vi "StartUp Sequence Open Loop Rev 1.5.vi"() -> ()   [LabVIEW 2017]
panel:
  out "Requested RPM":i32
  out "Waveform Chart":cluster{i32, i32}(graph)
  in  "Set RPM":string
  out "Pump Value 2":string
  in  "Soft Shut Off":bool
  out "Pump Value 1":string
  in  "Send RPM":bool
  in  "Send Command":bool
  in  "Custom Command":string
  out "Startup Success":bool
  in  "Output File":path
  in  "Shut Off":bool
  out "ECU COM Port Out":refnum<visa-resource-name>
  out "Throttle Position":string
  out "Turbine RPM":string
  out "Turbine Temp":string
  out "Error Out":errorcluster
  in  "Error In":errorcluster
  in  "ECU COM Port":refnum<visa-resource-name>
  out "Turbine State":string
  in  "Strt Sqnc":bool
  # "Note: save to a .csv file"
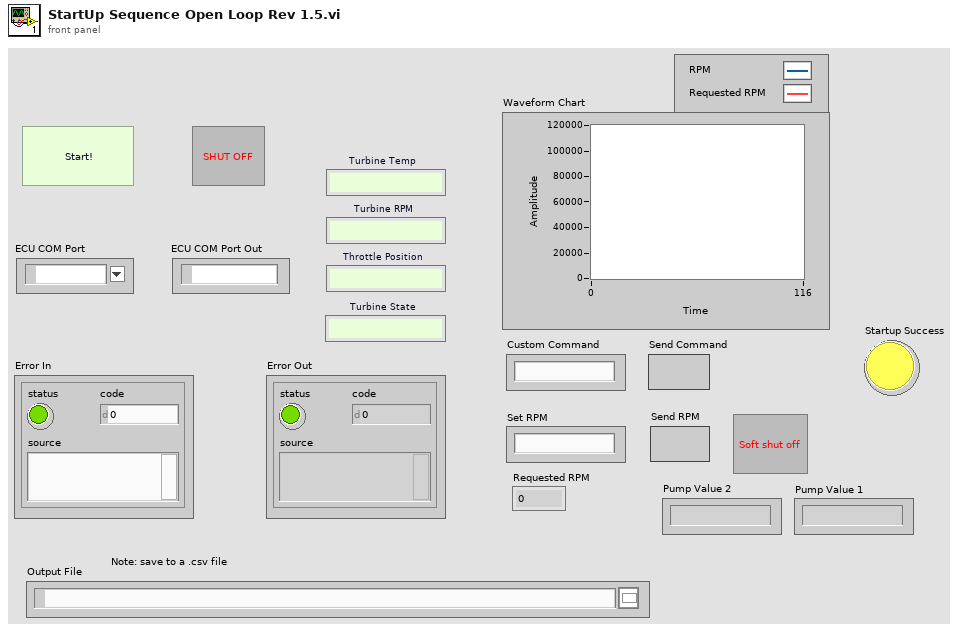
[diagram p1: front panel]
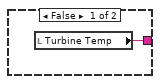
[diagram p4: hidden frame]
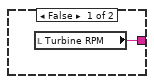
[diagram p5: hidden frame]
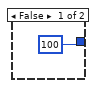
[diagram p7: hidden frame]
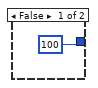
[diagram p8: hidden frame]
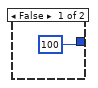
[diagram p9: hidden frame]
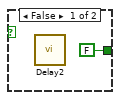
[diagram p11: hidden frame]
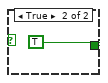
[diagram p12: hidden frame]
diagram:
  w15 = 21 ("Pulse Width")
  w16 = 160 ("Voltage")
  w21 = 16 ("Pulse Width")
  w22 = 160 ("Voltage")
  w12 = 255 ("y")
  w13 = 80 ("y")
  # "Disengage Starter Motor"
  # "Starter Motor 55%"
  # "Start button is inside a while loop that doesn't progess until True"
  # "Fuel Pump Mode 2"
  # "GlowPlugOff"
  # "Start Up\nFuelPumpMode 1"
  # "BurnerValveIgnitionPercent"
  # "If False, each Case structure is set\nto an arbitrary Delay time of 0.2 s"
  # "Each Stage is inside a while loop so that \nthe sequence doesn't progress until True"
  n1 = call "Initialize Com Port.vi"("Error In"="Error In", "ECU COM Port"="ECU COM Port") -> ("Error Out"=w36:errorcluster, "ECU COM Port Out"=w35:refnum<visa-resource-name>)  [unwired: 8 in]
  n2 = while {
    tunnel: w36 -> [w97]
    tunnel: [w97] -> w34
    stop <- "Strt Sqnc" stop-if-true
  }
  n3 = call "Initialize Output File.vi"("error in (no error)"=w34, "File Path Control"="Output File") -> ("error out"=w11:errorcluster)  [unwired: 9 in]
  n4 = flat-sequence {
    tunnel: w11 -> [w99]
    tunnel: [w99] -> w26
    frame #0 {
      n5 = local write "Strt Sqnc"(FALSE ("Strt Sqnc")) -> ()
    }
  }
  n6 = flat-sequence {
    tunnel: [w102] -> w10
    tunnel: w11 -> [w102]
    frame #0 {
      w101 = "0" ("Pump Value 1")
      n7 = local write "Pump Value 2"(w101) -> ()
      n8 = local write "Pump Value 1"(w101) -> ()
    }
  }
  n9 = while {
    tunnel: w10 -> [w123]
    tunnel: w35 -> [w122]
    tunnel: "Output File" -> [w119]
    stop <- w118 continue-if-true
    n10 = call "Get Engine Update.vi"("Error In"=w123, "ECU COM Port"=w122) -> ("Error Out"=w120:errorcluster, "Temperature"=w111:string, "RPMs"=w115:string, "ECU COM Port Out"=w117:refnum<visa-resource-name>)  [unwired: 6 in]
    n11 = call "Time Delay4"() -> ()  [unwired: 11 in, 1 out]
    n12 = call "Safety Check.vi"("Temperature"=w111, "RPMs"=w115) -> ("Safe?"=w118:bool)  [unwired: 9 in]
    n13 = Not Equal?(x=w115, y="") -> (x != y?=w113:bool)
    n14 = Not Equal?(x=w111, y="") -> (x != y?=w110:bool)
    n15 = case shown="False" w118 {
      selector: w118 -> [w128 w130]
      tunnel: w117 -> [w129 _]
      tunnel: [w128 w130] -> w116
      frame False {
        n16 = call "Emergency Shutoff.vi"("ECU COM Port"=w129) -> ()  [unwired: 9 in, 2 out]
      }
      frame True {
      }
    }
    n17 = case shown="True" w113 {
      tunnel: w115 -> [_ w127]
      tunnel: [w126 w127] -> w107
      frame False {
        n18 = local read "Turbine RPM"() -> (w126:string)
      }
      frame True {
        "Turbine RPM" <- w127
      }
    }
    n19 = case shown="True" w110 {
      tunnel: w111 -> [_ w125]
      tunnel: [w124 w125] -> w106
      frame False {
        n20 = local read "Turbine Temp"() -> (w124:string)
      }
      frame True {
        "Turbine Temp" <- w125
      }
    }
    n21 = Not(x=w116) -> (.not. x?=w121:bool)
    n22 = Stop(stop? (T)=w121) -> ()
    n23 = local read "Requested RPM"() -> (w104:i32)
    n24 = local read "Pump Value 2"() -> (w108:string)
    n25 = local read "Pump Value 1"() -> (w109:string)
    n26 = Decimal String To Number(string=w107) -> (number=w105:i32)  [unwired: 2 in, 1 out]
    n27 = Bundle(w105, "Requested RPM"=w104) -> (→"Waveform Chart":cluster{i32, "Requested RPM":i32})  [unwired: 1 in]
    n28 = call "Write Data to Output File.vi"("Pump Value 2"=w108, "Pump Value 1"=w109, "Error In"=w120, "Temperature"=w106, "RPM"=w107, "File Path Control"=w119) -> ()  [unwired: 5 in, 1 out]
  }
  n29 = while {
    tunnel: w35 -> [w132]
    tunnel: w36 -> [_]
    stop <- FALSE stop-if-true
    n30 = case shown="True" "Send Command" {
      tunnel: "Custom Command" -> [_ w136]
      tunnel: w132 -> [_ w135]
      frame False {
      }
      frame True {
        n31 = call "Time Delay3"() -> ()  [unwired: 11 in, 1 out]
        n32 = VISA Write(VISA resource name=w135, write buffer=w136) -> ()  [unwired: 1 in, 3 out]
      }
    }
  }
  n33 = flat-sequence {
    tunnel: w26 -> [_]
    frame #0 {
      n34 = local write "Turbine State"("Initializing Motor") -> ()
    }
  }
  n35 = while {
    tunnel: ["Shut Off"] -> w94
    tunnel: "ECU COM Port" -> [w138]
    stop <- "Shut Off" stop-if-true
    # "Turns off each individual component"
    n36 = case shown="True" "Shut Off" {
      tunnel: w138 -> [_ w142]
      frame False {
      }
      frame True {
        n37 = call "Emergency Shutoff.vi"("ECU COM Port"=w142) -> ("Error Out"=w141:errorcluster)  [unwired: 9 in, 1 out]
        n38 = local write "Output File"(path "" ("Output File")) -> ()
        n39 = flat-sequence {
          tunnel: w141 -> [w143]
          tunnel: [w143] -> _
          frame #0 {
            n40 = local write "Strt Sqnc"(FALSE ("Strt Sqnc")) -> ()
          }
        }
      }
    }
  }
  n41 = call "Set Glow Plug Duty Cycle.vi"("Error In"=w26, "Duty Cycle"=6, "ECU COM Port"=w35) -> ("Error Out"=w86:errorcluster, "ECU COM Port Out"=w83:refnum<visa-resource-name>)  [unwired: 7 in]
  n42 = call "Delay"("error in (no error)"=w86) -> ("error out"=w85:errorcluster)  [unwired: 10 in]
  n43 = call "Set Glow Plug Duty Cycle.vi"("Error In"=w85, "Duty Cycle"=19, "ECU COM Port"=w83) -> ("Error Out"=w84:errorcluster, "ECU COM Port Out"=w79:refnum<visa-resource-name>)  [unwired: 7 in]
  n44 = call "Delay"("error in (no error)"=w84) -> ("error out"=w80:errorcluster)  [unwired: 10 in]
  n45 = call "Set Starter Motor Duty Cycle.vi"("Error In"=w80, "Duty Cycle"=6, "ECU COM Port"=w79) -> ("Error Out"=w78:errorcluster, "ECU COM Port Out"=w76:refnum<visa-resource-name>)  [unwired: 7 in]
  n46 = call "Set Glow Plug Duty Cycle.vi"("Error In"=w78, "Duty Cycle"=15, "ECU COM Port"=w76) -> ("Error Out"=w77:errorcluster, "ECU COM Port Out"=w72:refnum<visa-resource-name>)  [unwired: 7 in]
  n47 = call "Delay"("error in (no error)"=w77) -> ("error out"=w74:errorcluster)  [unwired: 10 in]
  n48 = call "Set Starter Motor Duty Cycle.vi"("Error In"=w74, "Duty Cycle"=4, "ECU COM Port"=w72) -> ("Error Out"=w73:errorcluster, "ECU COM Port Out"=w71:refnum<visa-resource-name>)  [unwired: 7 in]
  n49 = call "Delay"("error in (no error)"=w73) -> ("error out"=w95:errorcluster)  [unwired: 10 in]
  n50 = Stop(stop? (T)=w94) -> ()
  n51 = while {
    tunnel: w95 -> [w147]
    tunnel: w71 -> [w146]
    tunnel: [w146] -> w24
    tunnel: [w147] -> w96
    stop <- w150 stop-if-true
    n52 = local read "Turbine RPM"() -> (w145:string)
    n53 = Decimal String To Number(string=w145) -> (number=w149:i32)  [unwired: 2 in, 1 out]
    n54 = Greater Or Equal?(x=w149, y=3300) -> (x >= y?=w151:bool)
    n55 = case shown="True" w151 {
      tunnel: [FALSE TRUE] -> w150
      frame False {
        n56 = call "Delay2"() -> ()  [unwired: 11 in, 1 out]
      }
      frame True {
      }
    }
  }
  n57 = flat-sequence {
    tunnel: w95 -> [_]
    frame #0 {
      n58 = local write "Turbine State"("Stage1 Check RPM") -> ()
    }
  }
  n59 = call "CmdSeparator7"("error in (no error)"=w96) -> ("error out"=w20:errorcluster)  [unwired: 10 in]
  n60 = call "Set Pump Fow Rate.vi"("Error In"=w20, "Pulse Width"=w21, "Voltage"=w22, "ECU COM Port"=w24) -> ("Error Out"=w25:errorcluster, "ECU COM Port Out"=w23:refnum<visa-resource-name>)  [unwired: 6 in]
  n61 = flat-sequence {
    tunnel: w22 -> [w156]
    tunnel: w21 -> [w155]
    tunnel: w20 -> [_]
    frame #0 {
      n62 = Number To Decimal String(number=w155) -> (decimal integer string=w157:string)  [unwired: 1 in]
      n63 = Number To Decimal String(number=w156) -> (decimal integer string=w158:string)  [unwired: 1 in]
      n64 = local write "Pump Value 2"(w157) -> ()
      n65 = local write "Pump Value 1"(w158) -> ()
    }
  }
  n66 = call "CmdSeparator2"("error in (no error)"=w25) -> ("error out"=w70:errorcluster)  [unwired: 10 in]
  n67 = call "Set Burner Valve Percent.vi"("Error In"=w70, "Percent"=10, "ECU COM Port"=w23) -> ("Error Out"=w69:errorcluster, "ECU COM Port Out"=w7:refnum<visa-resource-name>)  [unwired: 7 in]
  n68 = call "CmdSeparator"("error in (no error)"=w69) -> ("error out"=w6:errorcluster)  [unwired: 10 in]
  n69 = for {
    N: 8 -> [_]
    shift-right: [w164] -> _
    shift-left: 27 ("Percent") -> [w166]
    tunnel: w7 -> [w163]
    tunnel: w6 -> [w162]
    tunnel: [w160] -> w4
    tunnel: [w159] -> w3
    n70 = Add(x=w166, y=4 ("Percent")) -> (x+y=w164:i32)
    n71 = call "Set Burner Valve Percent.vi"("Error In"=w162, "Percent"=w164, "ECU COM Port"=w163) -> ("Error Out"=w161:errorcluster, "ECU COM Port Out"=w159:refnum<visa-resource-name>)  [unwired: 7 in]
    n72 = call "CmdSeparator4"("error in (no error)"=w161) -> ("error out"=w160:errorcluster)  [unwired: 10 in]
  }
  n73 = flat-sequence {
    tunnel: w4 -> [_]
    frame #0 {
      n74 = local write "Turbine State"("Stage2 Check Temp.") -> ()
    }
  }
  n75 = while {
    tunnel: [w168] -> _
    tunnel: w4 -> [w170]
    tunnel: [w168] -> w1
    tunnel: [w170] -> w2
    tunnel: w3 -> [w168]
    stop <- w173 stop-if-true
    # "Stage2Temp(C)"
    n76 = local read "Turbine Temp"() -> (w169:string)
    n77 = Decimal String To Number(string=w169) -> (number=w171:i32)  [unwired: 2 in, 1 out]
    n78 = Greater Or Equal?(x=w171, y=90) -> (x >= y?=w174:bool)
    n79 = case shown="False" w174 {
      tunnel: [FALSE TRUE] -> w173
      frame False {
        n80 = call "Delay3"() -> ()  [unwired: 11 in, 1 out]
      }
      frame True {
      }
    }
  }
  n81 = call "Set Glow Plug Duty Cycle.vi"("Error In"=w2, "Duty Cycle"=0, "ECU COM Port"=w1) -> ("Error Out"=w64:errorcluster, "ECU COM Port Out"=w17:refnum<visa-resource-name>)  [unwired: 7 in]
  n82 = call "CmdSeparator3"("error in (no error)"=w64) -> ("error out"=w14:errorcluster)  [unwired: 10 in]
  n83 = call "Set Pump Fow Rate.vi"("Error In"=w14, "Pulse Width"=w15, "Voltage"=w16, "ECU COM Port"=w17) -> ("Error Out"=w19:errorcluster, "ECU COM Port Out"=w18:refnum<visa-resource-name>)  [unwired: 6 in]
  n84 = call "Set Burner Valve Percent.vi"("Error In"=w19, "Percent"=80, "ECU COM Port"=w18) -> ("Error Out"=w61:errorcluster, "ECU COM Port Out"=w62:refnum<visa-resource-name>)  [unwired: 7 in]
  n85 = flat-sequence {
    tunnel: w16 -> [w178]
    tunnel: w15 -> [w177]
    tunnel: w14 -> [_]
    frame #0 {
      n86 = Number To Decimal String(number=w177) -> (decimal integer string=w179:string)  [unwired: 1 in]
      n87 = Number To Decimal String(number=w178) -> (decimal integer string=w180:string)  [unwired: 1 in]
      n88 = local write "Pump Value 2"(w179) -> ()
      n89 = local write "Pump Value 1"(w180) -> ()
    }
  }
  n90 = call "CmdSeparator18"("error in (no error)"=w61) -> ("error out"=w60:errorcluster)  [unwired: 10 in]
  n91 = call "Set Fuel Valve Percent.vi"("Error In"=w60, "Percent"=12, "ECU COM Port"=w62) -> ("Error Out"=w59:errorcluster, "ECU COM Port Out"=w63:refnum<visa-resource-name>)  [unwired: 7 in]
  n92 = call "CmdSeparator16"("error in (no error)"=w59) -> ("error out"=w92:errorcluster)  [unwired: 10 in]
  n93 = for {
    N: 4 -> [_]
    tunnel: [w181] -> _
    tunnel: [w195] -> _
    tunnel: w63 -> [w187]
    tunnel: w92 -> [w188]
    shift-right: [w186] -> w55
    shift-left: 12 -> [w192]
    shift-right: [w183] -> _
    shift-left: 80 -> [w189]
    tunnel: [w195] -> w50 mode=indexing
    tunnel: [w181] -> w56 mode=indexing
    n94 = Less?(x=w192, y=100) -> (x < y?=w193:bool)
    n95 = Less?(x=w189, y=100) -> (x < y?=w190:bool)
    n96 = case shown="True" w190 {
      tunnel: w189 -> [_ w199]
      tunnel: [100 w197] -> w183
      frame False {
      }
      frame True {
        n97 = Add(x=w199, y=5) -> (x+y=w197:i32)
      }
    }
    n98 = case shown="True" w193 {
      tunnel: w192 -> [_ w203]
      tunnel: [100 w201] -> w186
      frame False {
      }
      frame True {
        n99 = Add(x=w203, y=6) -> (x+y=w201:i32)
      }
    }
    n100 = call "Set Fuel Valve Percent.vi"("Error In"=w188, "Percent"=w186, "ECU COM Port"=w187) -> ("Error Out"=w185:errorcluster, "ECU COM Port Out"=w182:refnum<visa-resource-name>)  [unwired: 7 in]
    n101 = call "Set Burner Valve Percent.vi"("Error In"=w185, "Percent"=w183, "ECU COM Port"=w182) -> ("Error Out"=w184:errorcluster, "ECU COM Port Out"=w181:refnum<visa-resource-name>)  [unwired: 7 in]
    n102 = call "CmdSeparator17"("error in (no error)"=w184) -> ("error out"=w195:errorcluster)  [unwired: 10 in]
  }
  n103 = flat-sequence {
    tunnel: w50 -> [_]
    frame #0 {
      n104 = local write "Turbine State"("Pump Ramp Up") -> ()
    }
  }
  n105 = for {
    N: 10 -> [_]
    tunnel: [w211] -> w38
    tunnel: [w222] -> w41
    shift-right: [w218] -> _
    shift-left: w55 -> [w219]
    tunnel: w50 -> [w215] mode=indexing
    tunnel: w56 -> [w214] mode=indexing
    shift-right: [w207] -> w52
    shift-left: 21 -> [w208]
    w206 = 160 ("y")
    n106 = Less?(x=w219, y=100) -> (x < y?=w220:bool)
    n107 = Add(x=w208, y=1) -> (x+y=w207:i32)
    n108 = case shown="True" w220 {
      tunnel: w219 -> [_ w230]
      tunnel: [100 w228] -> w218
      frame False {
      }
      frame True {
        n109 = Add(x=w230, y=5) -> (x+y=w228:i32)
      }
    }
    n110 = call "Set Fuel Valve Percent.vi"("Error In"=w215, "Percent"=w218, "ECU COM Port"=w214) -> ("Error Out"=w217:errorcluster, "ECU COM Port Out"=w216:refnum<visa-resource-name>)  [unwired: 7 in]
    n111 = call "Set Burner Valve Percent.vi"("Error In"=w217, "Percent"=100 ("y"), "ECU COM Port"=w216) -> ("Error Out"=w205:errorcluster, "ECU COM Port Out"=w212:refnum<visa-resource-name>)  [unwired: 7 in]
    n112 = call "Set Pump Fow Rate.vi"("Error In"=w205, "Pulse Width"=w207, "Voltage"=w206, "ECU COM Port"=w212) -> ("Error Out"=w210:errorcluster, "ECU COM Port Out"=w211:refnum<visa-resource-name>)  [unwired: 6 in]
    n113 = flat-sequence {
      tunnel: w206 -> [w224]
      tunnel: w207 -> [w223]
      tunnel: w205 -> [_]
      frame #0 {
        n114 = Number To Decimal String(number=w223) -> (decimal integer string=w225:string)  [unwired: 1 in]
        n115 = Number To Decimal String(number=w224) -> (decimal integer string=w226:string)  [unwired: 1 in]
        n116 = local write "Pump Value 2"(w225) -> ()
        n117 = local write "Pump Value 1"(w226) -> ()
      }
    }
    n118 = call "CmdSeparator20"("error in (no error)"=w210) -> ("error out"=w222:errorcluster)  [unwired: 10 in]
  }
  n119 = call "Set Starter Motor Duty Cycle.vi"("Error In"=w41, "Duty Cycle"=11, "ECU COM Port"=w38) -> ("Error Out"=w40:errorcluster, "ECU COM Port Out"=w39:refnum<visa-resource-name>)  [unwired: 7 in]
  n120 = flat-sequence {
    tunnel: w40 -> [_]
    frame #0 {
      n121 = local write "Turbine State"("Secondary Pump Ramp Up") -> ()
    }
  }
  n122 = for {
    N: 3 -> [_]
    tunnel: [w239] -> w51
    tunnel: [w246] -> w49
    tunnel: w40 -> [w243]
    tunnel: w39 -> [w242]
    shift-right: [w233] -> _
    shift-left: w52 -> [w236]
    w234 = 160 ("y")
    n123 = Add(x=w236, y=10) -> (x+y=w233:i32)
    n124 = call "Set Fuel Valve Percent.vi"("Error In"=w243, "Percent"=100 ("y"), "ECU COM Port"=w242) -> ("Error Out"=w245:errorcluster, "ECU COM Port Out"=w244:refnum<visa-resource-name>)  [unwired: 7 in]
    n125 = call "Set Burner Valve Percent.vi"("Error In"=w245, "Percent"=0 ("y"), "ECU COM Port"=w244) -> ("Error Out"=w232:errorcluster, "ECU COM Port Out"=w240:refnum<visa-resource-name>)  [unwired: 7 in]
    n126 = call "Set Pump Fow Rate.vi"("Error In"=w232, "Pulse Width"=w233, "Voltage"=w234, "ECU COM Port"=w240) -> ("Error Out"=w238:errorcluster, "ECU COM Port Out"=w239:refnum<visa-resource-name>)  [unwired: 6 in]
    n127 = flat-sequence {
      tunnel: w234 -> [w248]
      tunnel: w233 -> [w247]
      tunnel: w232 -> [_]
      frame #0 {
        n128 = Number To Decimal String(number=w247) -> (decimal integer string=w249:string)  [unwired: 1 in]
        n129 = Number To Decimal String(number=w248) -> (decimal integer string=w250:string)  [unwired: 1 in]
        n130 = local write "Pump Value 2"(w249) -> ()
        n131 = local write "Pump Value 1"(w250) -> ()
      }
    }
    n132 = call "CmdSeparator15"("error in (no error)"=w238) -> ("error out"=w246:errorcluster)  [unwired: 10 in]
  }
  n133 = flat-sequence {
    tunnel: w49 -> [_]
    frame #0 {
      n134 = local write "Turbine State"("Hold on to your butts!") -> ()
    }
  }
  n135 = while {
    tunnel: w49 -> [w253]
    tunnel: w51 -> [w252]
    tunnel: [w253] -> w9
    tunnel: [w252] -> w48
    stop <- w254 stop-if-true
    n136 = local read "Turbine RPM"() -> (w257:string)
    n137 = Decimal String To Number(string=w257) -> (number=w256:i32)  [unwired: 2 in, 1 out]
    n138 = Greater?(x=w256, y=30000) -> (0:w254:bool)
  }
  n139 = call "Set Pump Fow Rate.vi"("Error In"=w9, "Pulse Width"=w12, "Voltage"=w13, "ECU COM Port"=w48) -> ("Error Out"=w47:errorcluster, "ECU COM Port Out"=w46:refnum<visa-resource-name>)  [unwired: 6 in]
  n140 = flat-sequence {
    tunnel: w13 -> [w260]
    tunnel: w12 -> [w259]
    tunnel: [w258] -> _
    tunnel: w9 -> [w258]
    frame #0 {
      n141 = Number To Decimal String(number=w259) -> (decimal integer string=w261:string)  [unwired: 1 in]
      n142 = Number To Decimal String(number=w260) -> (decimal integer string=w262:string)  [unwired: 1 in]
      n143 = local write "Pump Value 2"(w261) -> ()
      n144 = local write "Pump Value 1"(w262) -> ()
    }
  }
  n145 = while {
    tunnel: w47 -> [w264]
    tunnel: w46 -> [w263]
    tunnel: [w264] -> w43
    tunnel: [w263] -> w45
    stop <- w265 stop-if-true
    n146 = local read "Turbine RPM"() -> (w268:string)
    n147 = Decimal String To Number(string=w268) -> (number=w267:i32)  [unwired: 2 in, 1 out]
    n148 = Greater?(x=w267, y=44000) -> (0:w265:bool)
  }
  n149 = flat-sequence {
    tunnel: w43 -> [_]
    frame #0 {
      n150 = local write "Turbine State"("Acheived Idle RPM!") -> ()
    }
  }
  n151 = call "Set Starter Motor Duty Cycle.vi"("Error In"=w43, "Duty Cycle"=0, "ECU COM Port"=w45) -> ("Error Out"=w32:errorcluster, "ECU COM Port Out"=w31:refnum<visa-resource-name>)  [unwired: 7 in]
  n152 = flat-sequence {
    tunnel: w32 -> [_]
    frame #0 {
      "Startup Success" <- TRUE
    }
  }
  n153 = while {
    tunnel: w31 -> [w284]
    tunnel: [w283] -> w29
    tunnel: [w282] -> w30
    tunnel: w32 -> [w281]
    stop <- "Soft Shut Off" stop-if-true
    # "NOTE:\nThere are data entry limits\non this input. These may need\nto be deleted in the future"
    n154 = Decimal String To Number(string="Set RPM") -> (number=w272:i32)  [unwired: 2 in, 1 out]
    n155 = Less?(x=w272, y=135000) -> (x < y?=w278:bool)
    n156 = Greater?(x=w272, y=44000) -> (0:w273:bool)
    n157 = And(x=w273, y=w278) -> (x .and. y?=w276:bool)
    n158 = call "Time Delay"() -> ()  [unwired: 11 in, 1 out]
    n159 = And(x=w276, y="Send RPM") -> (x .and. y?=w274:bool)
    n160 = case shown="True" w274 {
      tunnel: w284 -> [w285 w295]
      tunnel: w281 -> [w286 w294]
      tunnel: [w285 w293] -> w283
      tunnel: [w286 w292] -> w282
      tunnel: w272 -> [_ w287]
      frame False {
      }
      frame True {
        n161 = call "RPM to Fuel Flow.vi"("Requested RPM"=w287) -> ("Fuel Pump Value 1"=w288:i32)  [unwired: 10 in]
        n162 = call "Set Pump Fow Rate.vi"("Error In"=w294, "Pulse Width"=255, "Voltage"=w288, "ECU COM Port"=w295) -> ("Error Out"=w292:errorcluster, "ECU COM Port Out"=w293:refnum<visa-resource-name>)  [unwired: 6 in]
        n163 = Number To Decimal String(number=w288) -> (decimal integer string=→"Pump Value 1":string)  [unwired: 1 in]
        n164 = local write "Pump Value 2"("255" ("Pump Value 2")) -> ()
        "Requested RPM" <- w287
      }
    }
  }
  n165 = call "Emergency Shutoff.vi"("Error In"=w30, "ECU COM Port"=w29) -> ("Error Out"=w28:errorcluster, "ECU COM Port Out"=→"ECU COM Port Out":refnum<visa-resource-name>)  [unwired: 8 in]
  n166 = flat-sequence {
    tunnel: w28 -> [w297]
    tunnel: [w297] -> w93
    frame #0 {
      w296 = "0"
      n167 = local write "Pump Value 1"(w296) -> ()
      n168 = local write "Pump Value 2"(w296) -> ()
    }
  }
  "Error Out" <- w93
